vi "VI-Change Runtime Menu Path.vi"(0 "Path":path, 5 "Old prefix":string="EPT", 7 "New prefix":string, 11 "error in (no error)":errorcluster) -> (15 "error out":errorcluster)   [LabVIEW 2020]
uses:
  <vilib>/regexp/Match Regular Expression.xnode
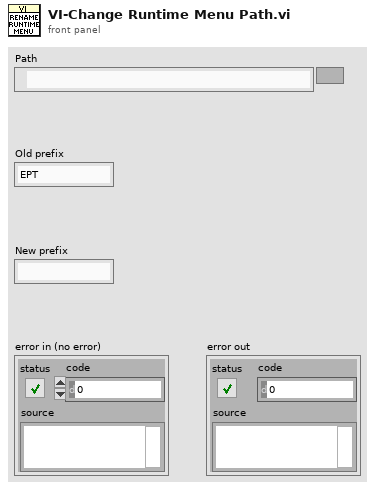
[diagram p1: front panel]
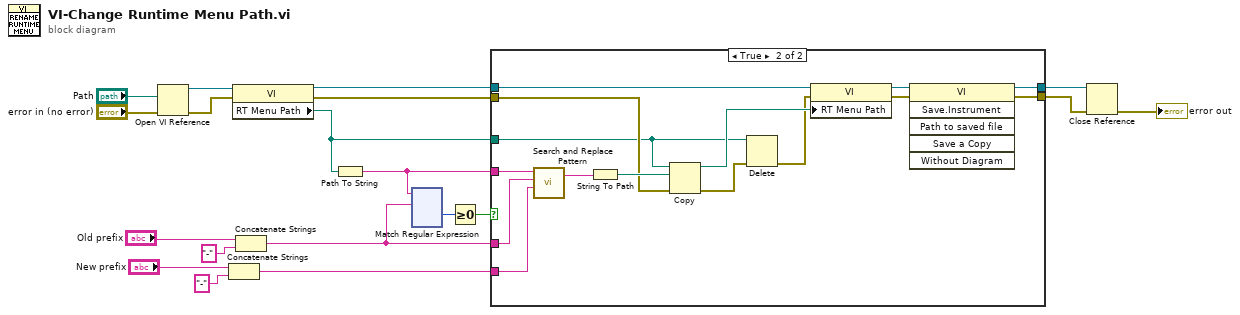
[diagram p0: block diagram]
diagram:
  n1 = Open VI Reference(vi path="Path", error in (no error)="error in (no error)") -> (vi reference=w6:refnum<vi>, error out=w5:errorcluster)  [unwired: 4 in]
  n2 = Concatenate Strings("New prefix", "-") -> (w13:string)
  n3 = property class="VI"(reference=w6, error in=w5) -> (reference out=w4:refnum<vi>, error out=w3:errorcluster, "RT Menu Path"=w2:path)
  n4 = Concatenate Strings("Old prefix", "-") -> (w12:string)
  n5 = Path To String(path=w2) -> (string=w7:string)
  n6 = xnode "Match Regular Expression"("input string"=w7, "regular expression"=w12) -> ("offset past match"=w8:i32)  [unwired: 4 in, 4 out]
  n7 = Greater Or Equal To 0?(x=w8) -> (x >= 0?=w1:bool)
  n8 = case shown="True" w1 {
    tunnel: w13 -> [_ w36]
    tunnel: w12 -> [_ w35]
    tunnel: [w21 w34] -> w11
    tunnel: [w20 w33] -> w10
    tunnel: w7 -> [_ w32]
    tunnel: w4 -> [w21 w30]
    tunnel: w3 -> [w20 w26]
    tunnel: w2 -> [_ w24]
    frame False {
    }
    frame True {
      n9 = call <vilib>:"Search and Replace Pattern.vi"("string"=w32, "regular expression (\"\")"=w35, "replace string (\"\")"=w36) -> ("result string"=w31:string)  [unwired: 2 in, 1 out]
      n10 = String To Path(string=w31) -> (path=w28:path)
      n11 = Copy(8:w26, 10:w28, 11:w24) -> (0:w25:errorcluster, 3:w27:path)  [unwired: 2 in, 1 out]
      n12 = Delete(path (use dialog)=w24, error in=w25) -> (error out=w23:errorcluster)  [unwired: 3 in, 2 out]
      n13 = property class="VI"(reference=w30, error in=w23, "RT Menu Path"=w27) -> (reference out=w29:refnum<vi>, error out=w22:errorcluster)
      n14 = invoke class="VI" method="Save.Instrument"(reference=w29, error in=w22) -> (reference out=w34:refnum<vi>, error out=w33:errorcluster)  [unwired: 4 in, 4 out]
    }
  }
  n15 = Close Reference(reference=w11, error in (no error)=w10) -> (error out=→"error out":errorcluster)
